vi "half cos gen.vi"() -> ()   [LabVIEW 2021]
uses:
  <vilib>/Analysis/1siggen.llb/Ramp Pattern by Samples.vi
  <vilib>/Analysis/NI_AALBase.lvlib
panel:
  out "Ramp Pattern":dbl[](array[numeric])
  out "Waveform Graph":dbl[](graph)
  out "Array":fxp<+/-,32,16>[](array[numeric])
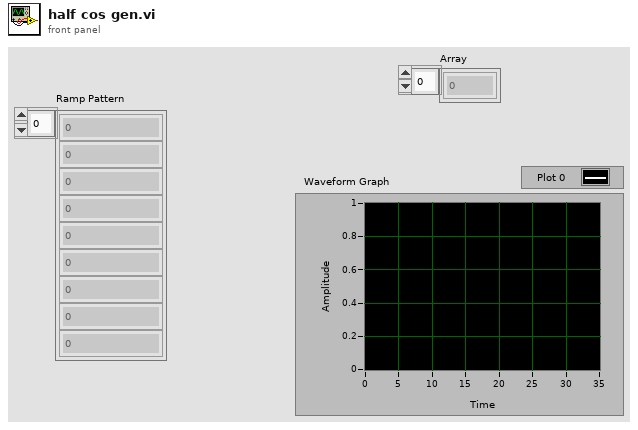
[diagram p1: front panel]
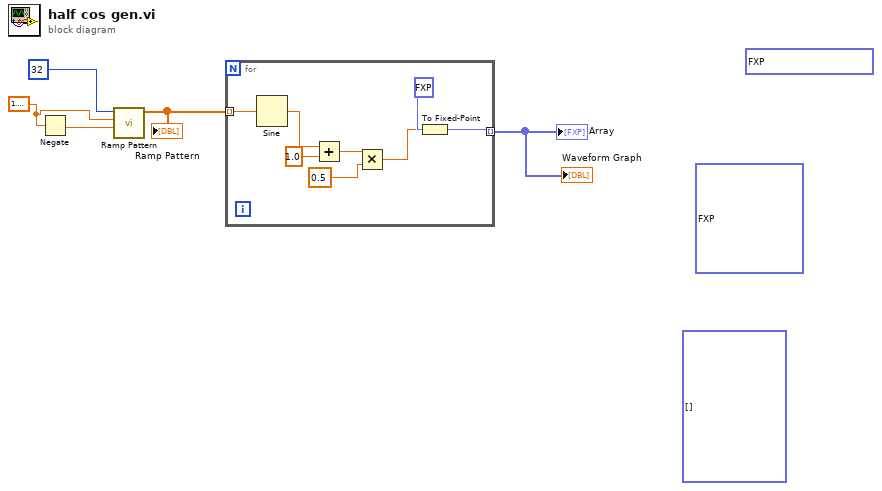
[diagram p0: block diagram]
diagram:
  (unwired) fxp<+/-,32,16>[] [0.0, 0.0025634765625, 0.0102386474609375, 0.0229339599609375, 0.04052734375, 0.0628204345703125, 0.0896148681640625, 0.1206207275390625, 0.155517578125, 0.1939544677734375, 0.2355194091796875, 0.2798004150390625, 0.32635498046875, 0.3746795654296875, 0.424285888671875, 0.47467041015625, 0.52532958984375, 0.575714111328125, 0.6253204345703125, 0.67364501953125, 0.7201995849609375, 0.7644805908203125, 0.8060455322265625, 0.844482421875, 0.8793792724609375, 0.9103851318359375, 0.9371795654296875, 0.95947265625, 0.9770660400390625, 0.9897613525390625, 0.9974365234375, 0.9999847412109375] ("Array 2")
  (unwired) fxp<+,16,0>[] []
  (unwired) fxp<+/-,32,16>[] [0.0, 0.000152587890625, 0.0006103515625, 0.001373291015625, 0.00244140625, 0.003814697265625, 0.0054931640625, 0.007476806640625, 0.009765625, 0.0123443603515625, 0.0152130126953125, 0.018402099609375, 0.0218658447265625, 0.025634765625, 0.0296783447265625, 0.034027099609375, 0.0386505126953125, 0.0435638427734375, 0.0487518310546875, 0.0542144775390625, 0.0599517822265625, 0.0659637451171875, 0.072235107421875, 0.078765869140625, 0.0855560302734375, 0.0926055908203125, 0.0998992919921875, 0.1074371337890625, 0.1152191162109375, 0.12322998046875, 0.1314849853515625, 0.13995361328125, 0.1486358642578125, 0.1575469970703125, 0.166656494140625, 0.1759796142578125, 0.1855010986328125, 0.1952056884765625, 0.205108642578125, 0.215179443359375, 0.225433349609375, 0.2358551025390625, 0.2464447021484375, 0.257171630859375, 0.26806640625, 0.279083251953125, 0.290252685546875, 0.301544189453125, 0.312957763671875, 0.3244781494140625, 0.3361053466796875, 0.34783935546875, 0.35968017578125, 0.37158203125, 0.383575439453125, 0.3956451416015625, 0.4077606201171875, 0.419952392578125, 0.43218994140625, 0.4444580078125, 0.4567718505859375, 0.4691009521484375, 0.4814453125, 0.4938201904296875, 0.5061798095703125, 0.5185546875, 0.5308990478515625, 0.5432281494140625, 0.5555419921875, 0.56781005859375, 0.580047607421875, 0.5922393798828125, 0.6043548583984375, 0.616424560546875, 0.62841796875, 0.64031982421875, 0.65216064453125, 0.6638946533203125, 0.6755218505859375, 0.687042236328125, 0.698455810546875, 0.709747314453125, 0.720916748046875, 0.73193359375, 0.742828369140625, 0.7535552978515625, 0.7641448974609375, 0.774566650390625, 0.784820556640625, 0.794891357421875, 0.8047943115234375, 0.8144989013671875, 0.8240203857421875, 0.833343505859375, 0.8424530029296875, 0.8513641357421875, 0.86004638671875, 0.8685150146484375, 0.87677001953125, 0.8847808837890625, 0.8925628662109375, 0.9001007080078125, 0.9073944091796875, 0.9144439697265625, 0.921234130859375, 0.927764892578125, 0.9340362548828125, 0.9400482177734375, 0.9457855224609375, 0.9512481689453125, 0.9564361572265625, 0.9613494873046875, 0.965972900390625, 0.9703216552734375, 0.974365234375, 0.9781341552734375, 0.981597900390625, 0.9847869873046875, 0.9876556396484375, 0.990234375, 0.992523193359375, 0.9945068359375, 0.996185302734375, 0.99755859375, 0.998626708984375, 0.9993896484375, 0.999847412109375, 0.9999847412109375] ("Array")
  w4 = 1.5707963267948966
  n1 = Negate(x=w4) -> (-x=w5:dbl)
  n2 = call-poly <vilib>:"Ramp Pattern.vi"("start"=w5, "end"=w4, "samples"=32) -> ("Ramp Pattern"=w2:dbl[])  [unwired: 7 in, 1 out]
  "Ramp Pattern" <- w2
  n3 = for {
    tunnel: w2 -> [w13] mode=indexing
    tunnel: [w12] -> w1 mode=indexing
    n4 = Sine(x=w13) -> (sin(x)=w10:dbl)
    n5 = Add(x=w10, y=1.0) -> (x+y=w8:dbl)
    n6 = Multiply(x=w8, y=0.5) -> (x*y=w6:dbl)
    n7 = To Fixed-Point(fixed-point type=fxp<+,16,0> 0.0, number=w6) -> (fixed-point=w12:fxp<+,16,0>)
  }
  "Array" <- w1
  "Waveform Graph" <- w1
